vi "SDSU_Dac_Check_Range.vi"(5 "resolution":i32=4095, 7 "unit":string, 8 "error in (no error)":errorcluster, 9 "value in":string, 10 "DACS":string[][](table), 11 "dac number":i32) -> (0 "error out":errorcluster, 1 "volts value":string, 2 "dac value":string, 4 "above range":bool, 6 "below range":bool)   [LabVIEW 2016]
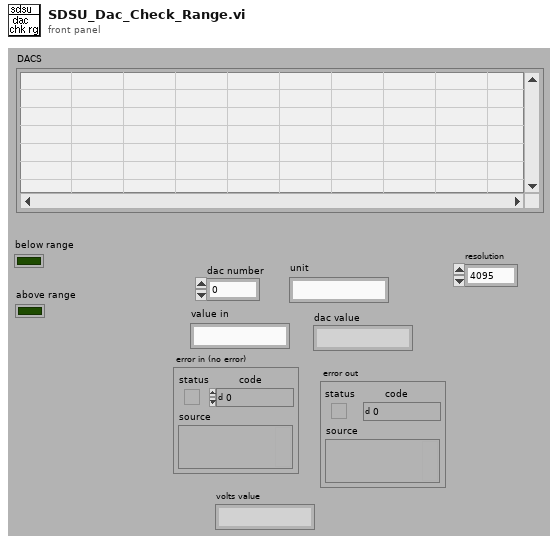
[diagram p1: front panel]
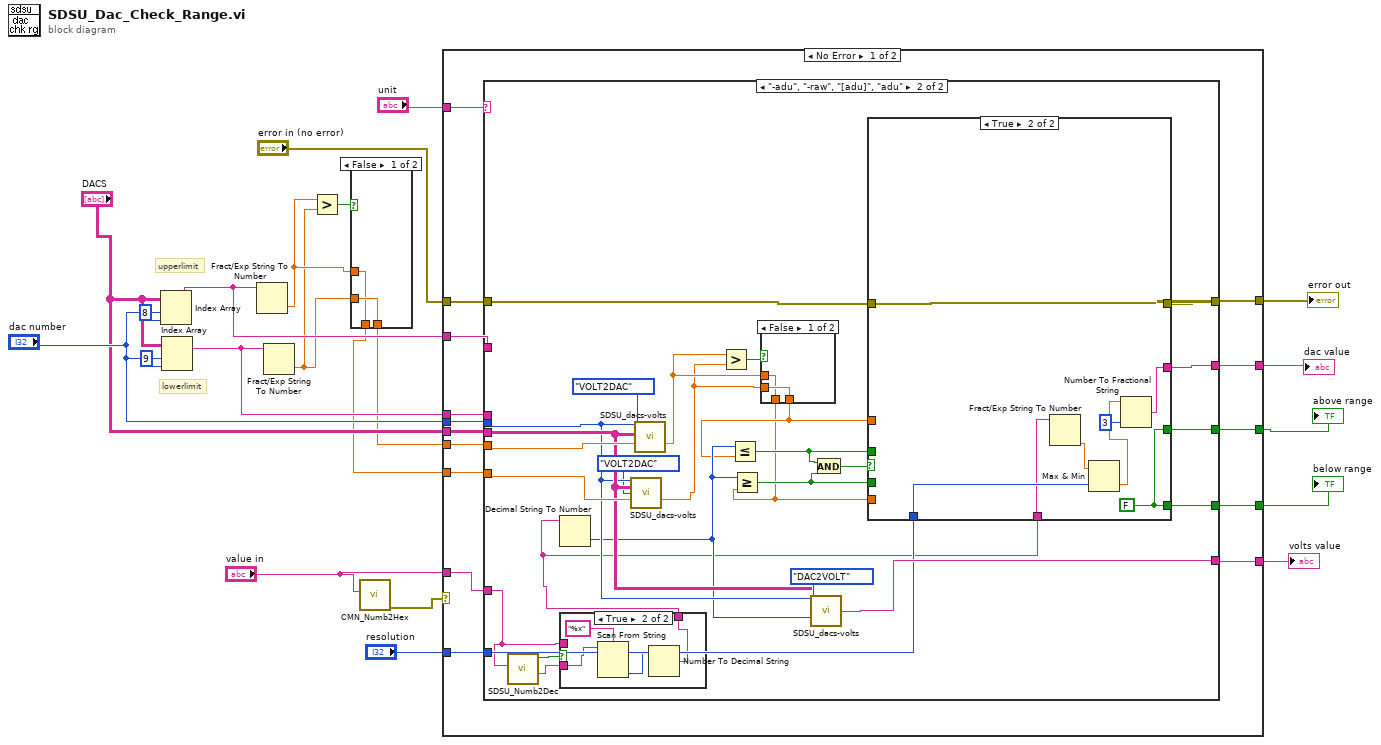
[diagram p0: block diagram]
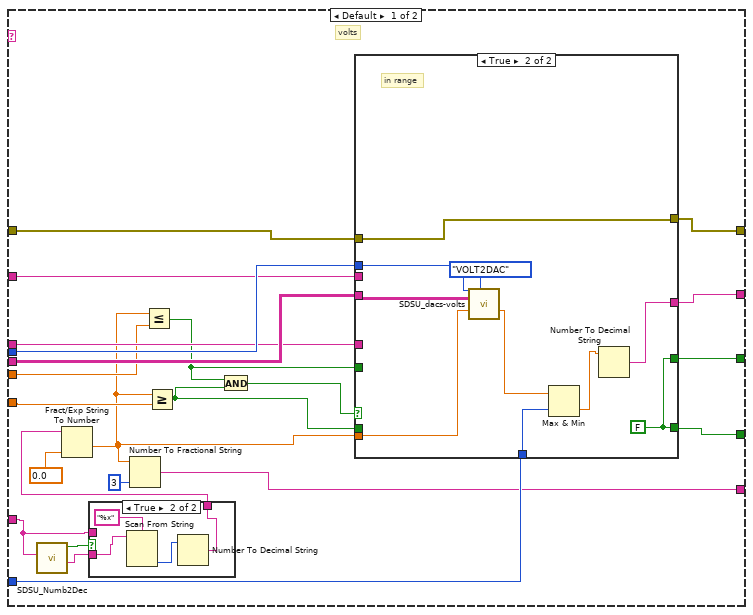
[diagram p3: hidden frame]
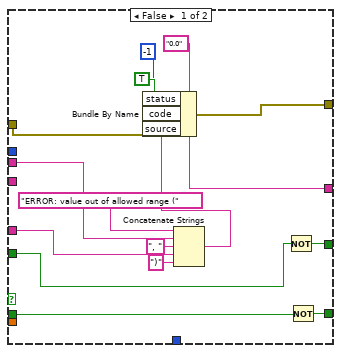
[diagram p5: hidden frame]
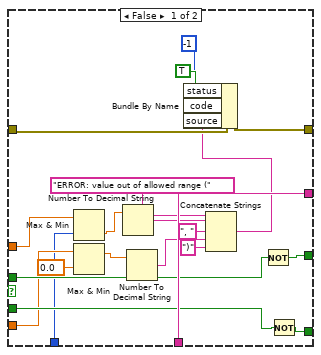
[diagram p8: hidden frame]
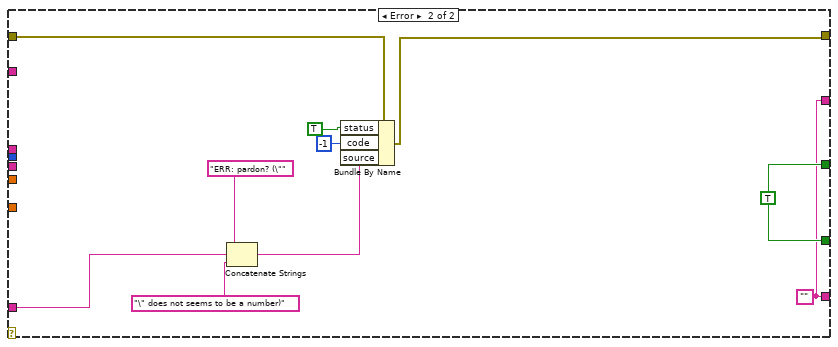
[diagram p9: hidden frame]
diagram:
  # "lowerlimit"
  # "upperlimit"
  n1 = Index Array(array="DACS", index (row)="dac number", index (col)=8 ("index (row)")) -> (element=w11:string)
  n2 = Index Array(array="DACS", index (row)="dac number", index (col)=9 ("index (row)")) -> (element=w12:string)
  n3 = Fract/Exp String To Number(string=w11) -> (number=w4:dbl)  [unwired: 4 out]
  n4 = Fract/Exp String To Number(string=w12) -> (number=w2:dbl)  [unwired: 4 out]
  n5 = Greater?(x=w4, y=w2) -> (0:w5:bool)
  n6 = case shown="False" w5 {
    tunnel: w4 -> [w22 w25]
    tunnel: [w23 w25] -> w3
    tunnel: w2 -> [w23 w24]
    tunnel: [w22 w24] -> w1
    frame False {
    }
    frame True {
    }
  }
  n7 = call "CMN_Numb2Hex.vi"("input str"="value in") -> ("error"=w6:errorcluster)  [unwired: 10 out]
  n8 = case shown="No Error" w6 {
    tunnel: "unit" -> [w40 _]
    tunnel: "error in (no error)" -> [w39 w166]
    tunnel: [w38 w165] -> w17
    tunnel: "dac number" -> [w37 _]
    tunnel: "DACS" -> [w36 _]
    tunnel: [w35 w163] -> w14
    tunnel: [w34 w163] -> w13
    tunnel: w12 -> [w33 _]
    tunnel: w11 -> [w32 _]
    tunnel: w1 -> [w31 _]
    tunnel: w3 -> [w30 _]
    tunnel: "resolution" -> [w29 _]
    tunnel: [w28 w164] -> w9
    tunnel: [w27 w164] -> w8
    tunnel: "value in" -> [w26 w161]
    frame No Error {
      n9 = case shown="\"-adu\", \"-raw\", \"[adu]\", \"adu\"" w40 {
        tunnel: w30 -> [w56 w119]
        tunnel: w31 -> [w55 w118]
        tunnel: w39 -> [w63 w116]
        tunnel: [w62 w115] -> w38
        tunnel: [w61 w117] -> w35
        tunnel: [w47 w113] -> w34
        tunnel: w26 -> [w43 w102]
        tunnel: w37 -> [w59 w111]
        tunnel: w36 -> [w60 w112]
        tunnel: w33 -> [w58 _]
        tunnel: w32 -> [w57 _]
        tunnel: w29 -> [w53 w108]
        tunnel: [w52 w107] -> w28
        tunnel: [w51 w106] -> w27
        frame Default {
          # "volts"
          n10 = call "SDSU_Numb2Dec.vi"("input str"=w43) -> ("output hexa"=w41:string, "hexa?"=w44:bool)  [unwired: 9 out]
          n11 = case shown="True" w44 {
            tunnel: w43 -> [w64 _]
            tunnel: [w64 w65] -> w42
            tunnel: w41 -> [_ w68]
            frame False {
            }
            frame True {
              n12 = Scan From String(format string="%x", input string=w68) -> (output 1=w66:u32)  [unwired: 2 in, 4 out]
              n13 = Number To Decimal String(number=w66) -> (decimal integer string=w65:string)  [unwired: 1 out]
            }
          }
          n14 = Fract/Exp String To Number(string=w42, default (0 dbl)=0.0) -> (number=w45:dbl)  [unwired: 3 out]
          n15 = Number To Fractional String(number=w45, precision (6)=i16 3) -> (F-format string=w47:string)  [unwired: 2 out]
          n16 = Less Or Equal?(x=w45, y=w56) -> (x <= y?=w49:bool)
          n17 = Greater Or Equal?(x=w45, y=w55) -> (x >= y?=w50:bool)
          n18 = And(x=w49, y=w50) -> (x .and. y?=w54:bool)
          n19 = case shown="True" w54 {
            tunnel: w63 -> [w82 w88]
            tunnel: [w80 w88] -> w62
            tunnel: w45 -> [_ w93]
            tunnel: w60 -> [_ w91]
            tunnel: w59 -> [_ w90]
            tunnel: ["0.0" w89] -> w61
            tunnel: w58 -> [w75 _]
            tunnel: w57 -> [w77 _]
            tunnel: w53 -> [_ w86]
            tunnel: [w69 w84] -> w52
            tunnel: [w70 w84] -> w51
            tunnel: w50 -> [w72 _]
            tunnel: w49 -> [w71 _]
            frame False {
              n20 = Concatenate Strings("ERROR: value out of allowed range (" ("source"), w77, ", " ("string"), w75, ")" ("string")) -> (w73:string)
              n21 = Bundle By Name(cluster=w82, "status"=TRUE, "code"=-1, "source"=w73) -> (w80:errorcluster)
              n22 = Not(x=w71) -> (.not. x?=w70:bool)
              n23 = Not(x=w72) -> (.not. x?=w69:bool)
            }
            frame True {
              w84 = FALSE
              # "in range"
              n24 = call "SDSU_dacs-volts.vi"("dac"=w90, "Table In"=w91, "action"=enum16{"DAC2VOLT", "VOLT2DAC"}."VOLT2DAC", "input value"=w93) -> ("output value"=w87:dbl)  [unwired: 11 out]
              n25 = Max & Min(x=w87, y=w86) -> (min(x,y)=w85:dbl)  [unwired: 1 out]
              n26 = Number To Decimal String(number=w85) -> (decimal integer string=w89:string)  [unwired: 1 out]
            }
          }
        }
        frame "-adu", "-raw", "[adu]", "adu" {
          n27 = call "SDSU_Numb2Dec.vi"("input str"=w102) -> ("output hexa"=w100:string, "hexa?"=w103:bool)  [unwired: 9 out]
          n28 = case shown="True" w103 {
            tunnel: w102 -> [w125 _]
            tunnel: [w125 w126] -> w101
            tunnel: w100 -> [_ w129]
            frame False {
            }
            frame True {
              n29 = Scan From String(format string="%x", input string=w129) -> (output 1=w127:u32)  [unwired: 2 in, 4 out]
              n30 = Number To Decimal String(number=w127) -> (decimal integer string=w126:string)  [unwired: 1 out]
            }
          }
          n31 = Decimal String To Number(string=w101) -> (number=w109:i32)  [unwired: 3 out]
          n32 = call "SDSU_dacs-volts.vi"("dac"=w111, "Table In"=w112, "action"=enum16{"DAC2VOLT", "VOLT2DAC"}."VOLT2DAC", "input value"=w118) -> ("output value"=w96:dbl)  [unwired: 11 out]
          n33 = call "SDSU_dacs-volts.vi"("dac"=w111, "Table In"=w112, "action"=enum16{"DAC2VOLT", "VOLT2DAC"}."VOLT2DAC", "input value"=w119) -> ("output value"=w98:dbl)  [unwired: 11 out]
          n34 = Greater?(x=w98, y=w96) -> (0:w99:bool)
          n35 = case shown="False" w99 {
            tunnel: w98 -> [w121 w124]
            tunnel: [w122 w124] -> w97
            tunnel: w96 -> [w122 w123]
            tunnel: [w121 w123] -> w95
            frame False {
            }
            frame True {
            }
          }
          n36 = Less Or Equal?(x=w109, y=w97) -> (x <= y?=w105:bool)
          n37 = Greater Or Equal?(x=w109, y=w95) -> (x >= y?=w104:bool)
          n38 = call "SDSU_dacs-volts.vi"("dac"=w111, "Table In"=w112, "action"=enum16{"DAC2VOLT", "VOLT2DAC"}."DAC2VOLT", "input value"=w109) -> ("string value"=w113:string)  [unwired: 11 out]
          n39 = And(x=w105, y=w104) -> (x .and. y?=w94:bool)
          n40 = case shown="True" w94 {
            tunnel: w101 -> [w150 w154]
            tunnel: [w150 w153] -> w117
            tunnel: w116 -> [w147 w158]
            tunnel: [w146 w158] -> w115
            tunnel: w108 -> [w131 w157]
            tunnel: [w138 w151] -> w107
            tunnel: [w141 w151] -> w106
            tunnel: w105 -> [w140 _]
            tunnel: w104 -> [w139 _]
            tunnel: w97 -> [w137 _]
            tunnel: w95 -> [w134 _]
            frame False {
              n41 = Max & Min(x=w137, y=w131) -> (min(x,y)=w136:dbl)  [unwired: 1 out]
              n42 = Max & Min(x=w134, y=0.0) -> (max(x,y)=w133:dbl)  [unwired: 1 out]
              n43 = Number To Decimal String(number=w136) -> (decimal integer string=w135:string)  [unwired: 1 out]
              n44 = Number To Decimal String(number=w133) -> (decimal integer string=w132:string)  [unwired: 1 out]
              n45 = Concatenate Strings("ERROR: value out of allowed range (" ("source"), w135, ", " ("string"), w132, ")" ("string")) -> (w142:string)
              n46 = Bundle By Name(cluster=w147, "status"=TRUE, "code"=-1, "source"=w142) -> (w146:errorcluster)
              n47 = Not(x=w140) -> (.not. x?=w141:bool)
              n48 = Not(x=w139) -> (.not. x?=w138:bool)
            }
            frame True {
              w151 = FALSE
              n49 = Fract/Exp String To Number(string=w154) -> (number=w156:dbl)  [unwired: 4 out]
              n50 = Max & Min(x=w156, y=w157) -> (min(x,y)=w155:dbl)  [unwired: 1 out]
              n51 = Number To Fractional String(number=w155, precision (6)=i16 3) -> (F-format string=w153:string)  [unwired: 2 out]
            }
          }
        }
      }
    }
    frame Error {
      w164 = TRUE
      w163 = ""
      n52 = Concatenate Strings("ERR: pardon? (\"" ("source"), w161, "\" does not seems to be a number)" ("string")) -> (w159:string)
      n53 = Bundle By Name(cluster=w166, "status"=TRUE, "code"=-1, "source"=w159) -> (w165:errorcluster)
    }
  }
  "error out" <- w17
  "dac value" <- w14
  "volts value" <- w13
  "above range" <- w8
  "below range" <- w9
